vi "Run Detection.vi"(4 "Specific target IP":string, 6 "Specific target (F)":bool, 7 "Reduce Discovery Timeout (T)":bool=TRUE, 8 "error in (no error)":errorcluster, 10 "Targets in":T2 {"Filtered Targets"."IP Mode" items=["Static"=1, "DHCP/Link-Local"=2, "Link-Local Only"=4, "DHCP Only"=8]}, 11 "Ctl Refs in":T5) -> (0 "error out":errorcluster, 1 "State":T1, 2 "Targets out":T2 {"Filtered Targets"."IP Mode" items=["Static"=1, "DHCP/Link-Local"=2, "Link-Local Only"=4, "DHCP Only"=8]}, 3 "Ctl Refs out":T5)   [LabVIEW 2013]
uses:
  Controls/Refs.ctl
  Controls/Button Refs.ctl
  Controls/Tab Ctl Refs.ctl
  types/TabStateType.ctl
  Controls/Indicator Refs.ctl
  Controls/Slider Refs.ctl
  Controls/Control Refs.ctl
  Controls/Targets.ctl
  Controls/Detected.ctl
  types/MAX Sys Cfg Target Information.ctl
  types/ExecutionStateType.ctl
panel:
  in  "stop":bool
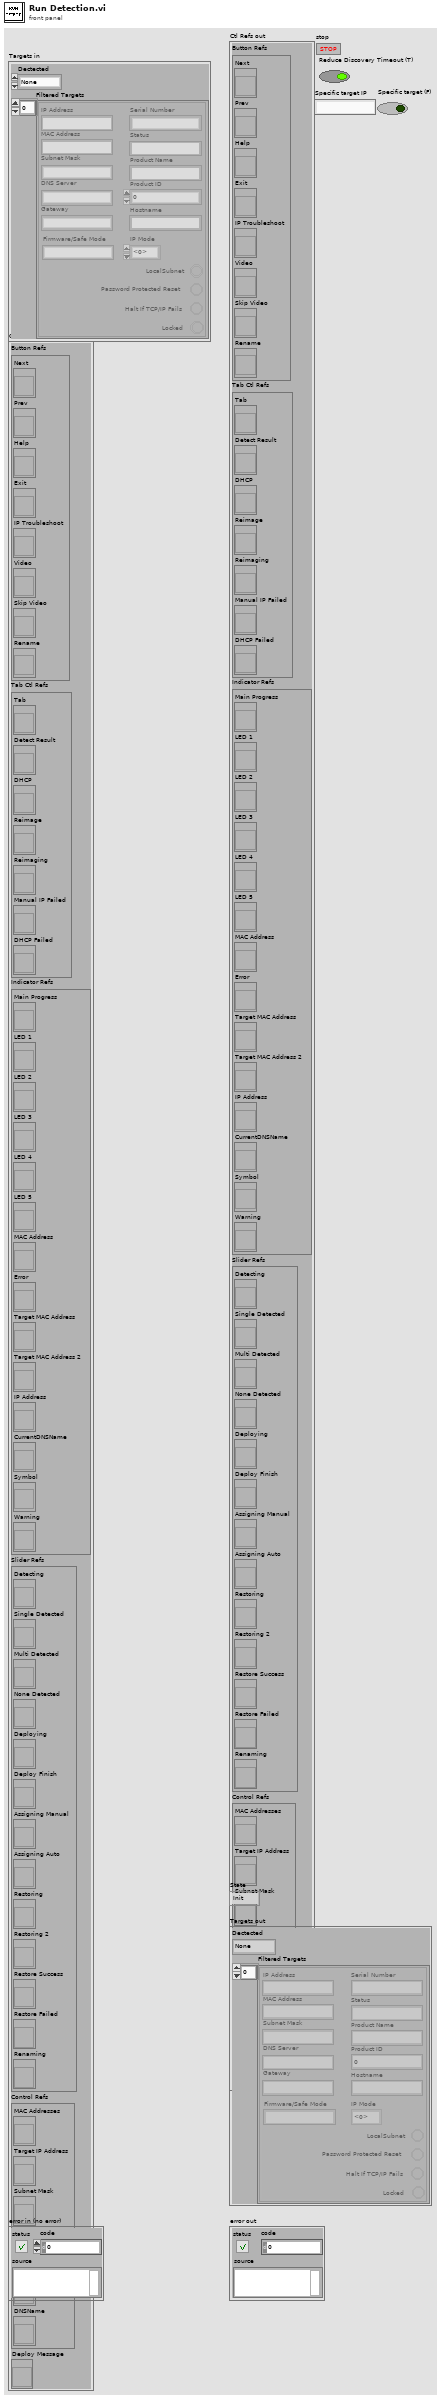
[diagram p1: front panel]
types:
  T1 = typedef "ExecutionStateType.ctl" = enum16{"Init", "Welcome", "Idle", "Detect", "Run Detection", "Detect Fail", "Detect One", "Detect Mult", "Deploy", "DHCP", "Static IP", "Run Deployment", "Connect Verify", "Exit", "Video Wait", "Success", "Troubleshoot", "Troubleshoot 2", "RenameDNS"}
  T2 = typedef "Targets.ctl" = cluster{"Dectected":T3, "Filtered Targets":T4[]}
  T3 = typedef "Detected.ctl" = enum16{"None", "Failed", "Single", "Multi"}
  T4 = typedef "MAX Sys Cfg Target Information.ctl" = cluster{"MAC Address":string, "IP Address":string, "Status":string, "Product Name":string, "Hostname":string, "Firmware/Safe Mode":string, "Subnet Mask":string, "Gateway":string, "DNS Server":string, "Serial Number":string, "Product ID":u32, "Locked ":bool, "LocalSubnet":bool, "Halt If TCP/IP Fails":bool, "Password Protected Reset":bool, "IP Mode":i32}
  T5 = typedef "Refs.ctl" = cluster{"Button Refs":T6, "Tab Ctl Refs":T7, "Indicator Refs":T8, "Slider Refs":T9, "Control Refs":T10, "Deploy Message":refnum<vi>}
  T6 = typedef "Button Refs.ctl" = cluster{"Next":refnum<vi>, "Prev":refnum<vi>, "Help":refnum<vi>, "Exit":refnum<vi>, "IP Troubleshoot":refnum<vi>, "Video":refnum<vi>, "Skip Video":refnum<vi>, "Rename":refnum<vi>}
  T7 = typedef "Tab Ctl Refs.ctl" = cluster{"Tab":refnum<vi>, "Detect Result":refnum<vi>, "DHCP":refnum<vi>, "Reimage":refnum<vi>, "Reimaging":refnum<vi>, "Manual IP Failed":refnum<vi>, "DHCP Failed":refnum<vi>}
  T8 = typedef "Indicator Refs.ctl" = cluster{"Main Progress":refnum<vi>, "LED 1":refnum<vi>, "LED 2":refnum<vi>, "LED 3":refnum<vi>, "LED 4":refnum<vi>, "LED 5":refnum<vi>, "MAC Address":refnum<vi>, "Error":refnum<vi>, "Target MAC Address":refnum<vi>, "Target MAC Address 2":refnum<vi>, "IP Address":refnum<vi>, "CurrentDNSName":refnum<vi>, "Symbol":refnum<vi>, "Warning":refnum<vi>}
  T9 = typedef "Slider Refs.ctl" = cluster{"Detecting":refnum<vi>, "Single Detected":refnum<vi>, "Multi Detected":refnum<vi>, "None Detected":refnum<vi>, "Deploying":refnum<vi>, "Deploy Finish":refnum<vi>, "Assigning Manual":refnum<vi>, "Assigning Auto":refnum<vi>, "Restoring":refnum<vi>, "Restoring 2":refnum<vi>, "Restore Success":refnum<vi>, "Restore Failed":refnum<vi>, "Renaming":refnum<vi>}
  T10 = typedef "Control Refs.ctl" = cluster{"MAC Addresses":refnum<vi>, "Target IP Address":refnum<vi>, "Subnet Mask":refnum<vi>, "DNS IP":refnum<vi>, "Default Gateway":refnum<vi>, "DNSName":refnum<vi>}
  T11 = enum32{"Welcome", "Instructions", "Detect", "Run Detection", "Detect Result", "Deploy", "Run Deployment", "Connect Verify", "Success", "DHCP", "Troubleshoot", "System Restore"}
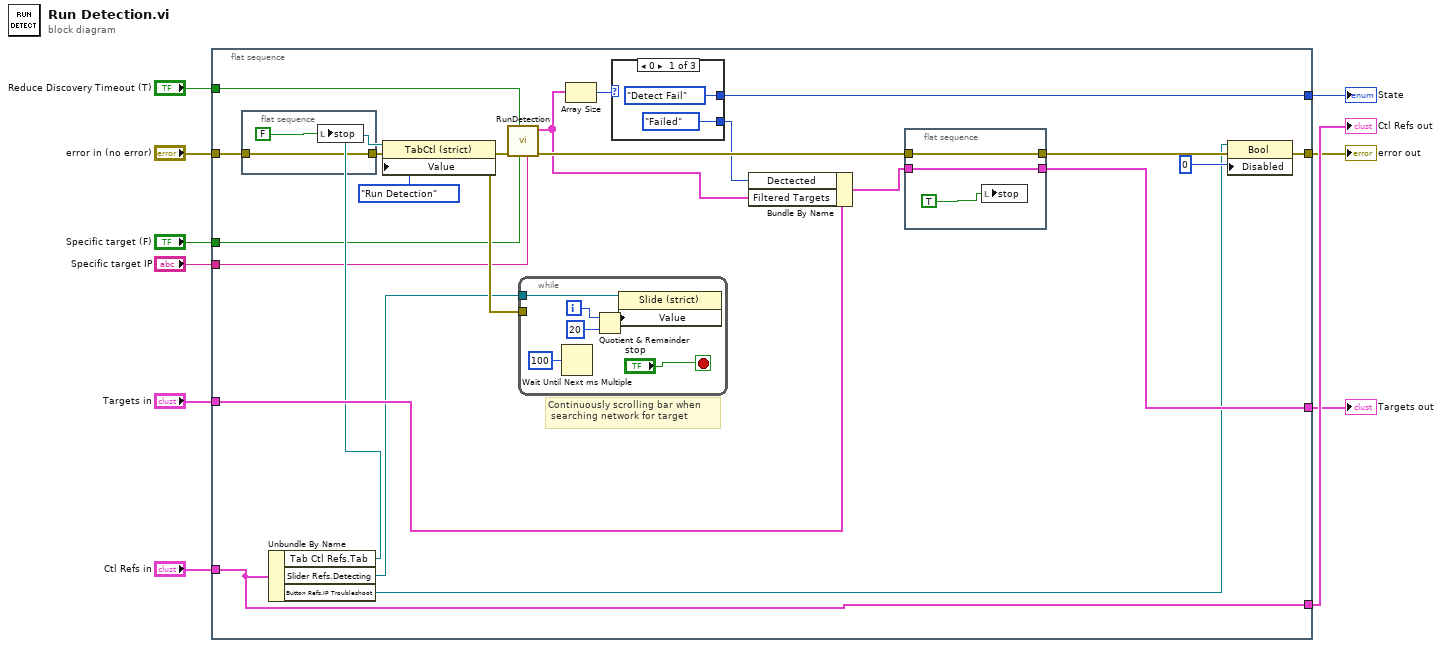
[diagram p0: block diagram]
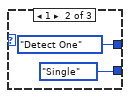
[diagram p2: hidden frame]
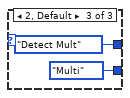
[diagram p3: hidden frame]
diagram:
  n1 = flat-sequence {
    tunnel: [w32] -> w4
    tunnel: [w30] -> w5
    tunnel: "error in (no error)" -> [w29]
    tunnel: [w25] -> w7
    tunnel: "Targets in" -> [w21]
    tunnel: "Ctl Refs in" -> [w14]
    tunnel: [w14] -> w10
    tunnel: "Reduce Discovery Timeout (T)" -> [w13]
    tunnel: "Specific target (F)" -> [w12]
    tunnel: "Specific target IP" -> [w11]
    frame #0 {
      # "Continuously scrolling bar when\n searching network for target"
      n2 = flat-sequence {
        tunnel: w29 -> [w40]
        tunnel: [w40] -> w28
        frame #0 {
          n3 = local write "stop"(FALSE) -> ()
        }
      }
      n4 = Unbundle By Name(w14) -> ("Tab Ctl Refs.Tab"=w17:refnum<vi>, "Slider Refs.Detecting"=w15:refnum<vi>, "Button Refs.IP Troubleshoot"=w16:refnum<vi>)
      n5 = property on="Property Node" class="TabCtl (strict)"(reference=w17, error in=w28, "Value"=T11."Run Detection" ("Tab Control")) -> (error out=w22:errorcluster)  [unwired: 1 out]
      n6 = call "RunDetection.vi"("Specific target IP"=w11, "Specific target (F)"=w12, "Reduce discovery timeout (T)"=w13, "error in (no error)"=w22) -> ("error out"=w23:errorcluster, "Filtered Targets"=w19:T4[])  [unwired: 6 in]
      n7 = while {
        tunnel: w22 -> [_]
        tunnel: w15 -> [w34]
        i -> [w36]
        stop <- "stop" stop-if-true
        n8 = Wait Until Next ms Multiple(millisecond multiple=u32 100 ("milliseconds to wait")) -> ()  [unwired: 1 out]
        n9 = Quotient & Remainder(x=w36, y=20) -> (x-y*floor(x/y)=w35:i32)  [unwired: 1 out]
        n10 = property on="Property Node" class="Slide (strict)"(reference=w34, "Value"=w35) -> ()  [unwired: 1 in, 2 out]
      }
      n11 = Array Size(array=w19) -> (size(s)=w31:i32)
      n12 = case shown="0" w31 {
        tunnel: [ExecutionStateType."Detect Fail" ("Enum") ExecutionStateType."Detect One" ("Enum") ExecutionStateType."Detect Mult" ("Enum")] -> w32
        tunnel: [Detected."Failed" Detected."Single" Detected."Multi"] -> w20
        frame 0 {
        }
        frame 1 {
        }
        frame 2, Default {
        }
      }
      n13 = Bundle By Name(cluster=w21, "Dectected"=w20, "Filtered Targets"=w19) -> (w18:T2)
      n14 = flat-sequence {
        tunnel: [w42] -> w26
        tunnel: [w43] -> w30
        tunnel: w18 -> [w43]
        tunnel: w23 -> [w42]
        frame #0 {
          n15 = local write "stop"(TRUE) -> ()
        }
      }
      n16 = property on="Property Node" class="Bool"(reference=w16, error in=w26, "Disabled"=u8 0) -> (error out=w25:errorcluster)  [unwired: 1 out]
    }
  }
  "Ctl Refs out" <- w10
  "error out" <- w7
  "Targets out" <- w5
  "State" <- w4
